vi "p8.11.vi"() -> ()   [LabVIEW 2020]
uses:
  <vilib>/vision/NI_Vision_Development_Module.lvlib
panel:
  out "Waveform Graph":T1(graph)={"Starting Value"=0.0, "Incremental Value"=1.0, "Histogram"=[135, 232, 258, 257, 246, 246, 247, 251, 269, 242, 234, 244, 257, 253, 251, 246, 258, 238, 260, 257, 297, 264, 258, 234, 237, 230, 276, 260, 262, 256, 238, 280, 256, 256, 234, 245, 284, 260, 278, 270, 291, 231, 257, 254, 240, 231, 247, 270, 246, 268, 266, 245, 244, 274, 252, 259, 282, 240, 251, 240, 250, 247, 263, 242, 256, 258, 226, 285, 271, 269, 247, 231, 253, 245, 251, 279, 233, 254, 242, 280, 256, 255, 269, 260, 218, 235, 246, 247, 252, 240, 228, 242, 251, 264, 253, 269, 262, 267, 264, 260, 245, 256, 263, 267, 250, 248, 249, 278, 252, 252, 249, 262, 269, 245, 287, 274, 250, 265, 248, 242, 266, 244, 266, 274, 284, 255, 259, 255, 246, 246, 284, 268, 234, 287, 223, 267, 259, 257, 233, 298, 273, 276, 268, 259, 276, 257, 238, 281, 244, 259, 257, 255, 265, 242, 283, 286, 273, 251, 246, 270, 234, 254, 269, 245, 246, 228, 272, 251, 244, 270, 251, 260, 244, 259, 225, 260, 257, 269, 257, 258, 252, 263, 263, 255, 251, 286, 260, 277, 259, 255, 283, 257, 264, 239, 240, 267, 270, 264, 252, 268, 261, 282, 256, 246, 266, 273, 227, 270, 239, 270, 241, 264, 257, 246, 265, 267, 224, 260, 249, 263, 258, 263, 249, 239, 249, 278, 247, 265, 282, 265, 265, 266, 266, 247, 250, 255, 243, 256, 280, 239, 267, 266, 247, 264, 282, 291, 291, 275, 250, 249, 241, 248, 274, 264, 262, 120]}
  out "Ruido blanco":T2(plugin-control)
  in  "Valor maximo (Unsigned 16 bits)":u16=255
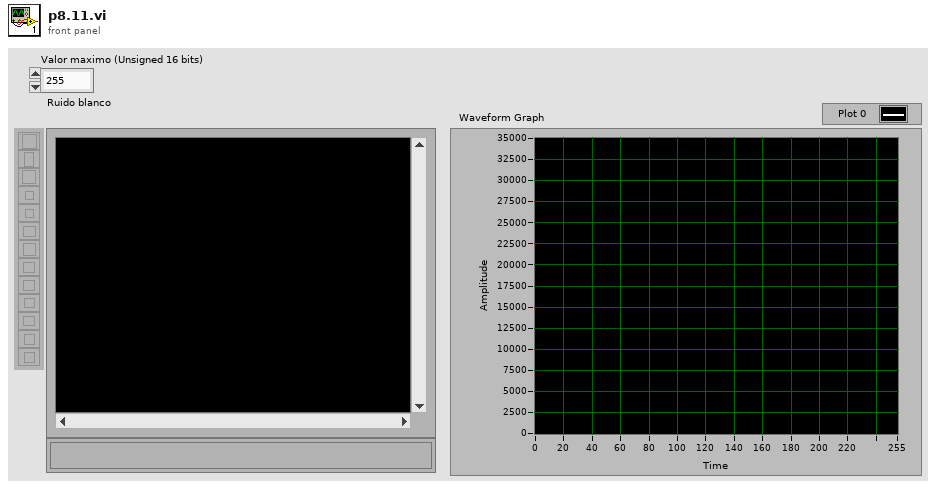
[diagram p1: front panel]
types:
  T1 = cluster{"Starting Value":sgl, "Incremental Value":sgl, "Histogram":u32[]}
  T2 = typedef "IMAQ Image.ctl" = refnum<image>
  T3 = typedef "Image Type" = u32
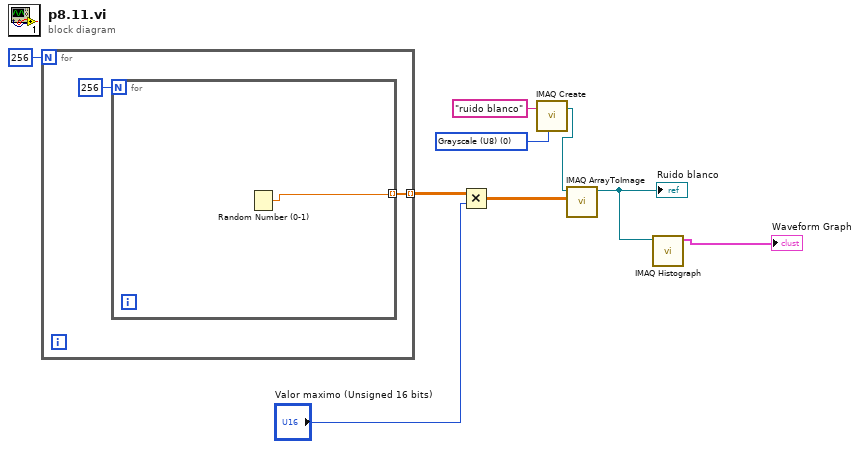
[diagram p0: block diagram]
diagram:
  w5 = T3 0 items=["Grayscale (U8)", "Grayscale (I16)", "Grayscale (SGL)", "Complex (CSG)", "RGB (U32)", "HSL (U32)", "RGB (U64)", "Grayscale (U16)"] ("Image Type")
  n1 = for {
    N: 256 -> [_]
    tunnel: [w10] -> w8 mode=indexing
    n2 = for {
      N: 256 -> [_]
      tunnel: [w12] -> w10 mode=indexing
      n3 = Random Number (0-1)() -> (number: 0 to 1=w12:dbl)
    }
  }
  n4 = Multiply(x=w8, y="Valor maximo (Unsigned 16 bits)") -> (x*y=w4:dbl[][])
  n5 = call "IMAQ Create"("Image Name"="ruido blanco", "Image Type"=w5) -> ("New Image"=w3:T2)  [unwired: 3 in, 1 out]
  n6 = call "IMAQ ArrayToImage"("Image Pixels (U8)"=w4, "Image"=w3) -> ("Image Out"=w2:T2)  [unwired: 8 in, 1 out]
  "Ruido blanco" <- w2
  n7 = call "IMAQ Histograph"("Image"=w2) -> ("Histogram Graph"=→"Waveform Graph":T1)  [unwired: 7 in, 3 out]
